vi "K_S30_VISA F30.vi"(4 "error in":errorcluster, 6 "Coeff. Nr.":u8=64, 7 "Address":u8=250) -> (0 "error out":errorcluster, 3 "Coeff":sgl format="%.6e")   [LabVIEW 2012]
panel:
  # "Function 30: Read coefficient\nV1.0, b.v."
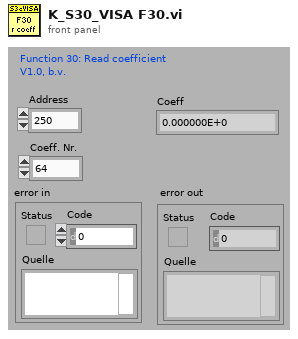
[diagram p1: front panel]
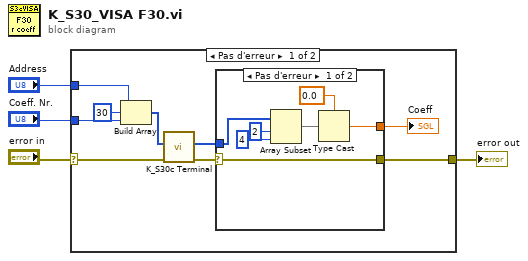
[diagram p0: block diagram]
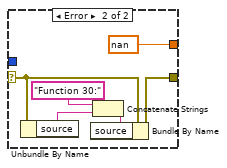
[diagram p2: hidden frame]
diagram:
  n1 = case shown="Pas d'erreur" "error in" {
    selector: "error in" -> [w10 w27]
    tunnel: "Address" -> [w13 _]
    tunnel: [w8 w27] -> w2
    tunnel: "Coeff. Nr." -> [w6 _]
    frame No Error {
      n2 = Build Array(w13, u8 30 ("Element"), w6) -> (w11:u8[])
      n3 = call "K_S30c Terminal.vi"("error in"=w10, "request"=w11) -> ("error out"=w9:errorcluster, "response"=w7:u8[])  [unwired: 4 in]
      n4 = case shown="Pas d'erreur" w9 {
        selector: w9 -> [w20 w26]
        tunnel: [w20 w24] -> w8
        tunnel: w7 -> [w19 _]
        tunnel: [w15 sgl nan] -> w5
        frame No Error {
          n5 = Array Subset(array=w19, index=2 ("Index"), length=4 ("Länge")) -> (w14:u8[])
          n6 = Type Cast(type=sgl 0.0, x=w14) -> (*(type *) &x=w15:sgl)
        }
        frame Error {
          n7 = Unbundle By Name(w26) -> ("source"=w22:string)
          n8 = Concatenate Strings("Function 30:" ("String"), w22) -> (w25:string)
          n9 = Bundle By Name(cluster=w26, "source"=w25) -> (w24:errorcluster)
        }
      }
      "Coeff" <- w5
    }
    frame Error {
    }
  }
  "error out" <- w2
